vi "Untitled 1.vi"() -> ()   [LabVIEW 2010]
uses:
  <vilib>/MDSplus/Classes/Data_Class/Array_Class/Array.lvclass
  <vilib>/MDSplus/Classes/Data_Class/Array_Class/Float32Array_Class/Float32Array.lvclass
  <vilib>/MDSplus/Classes/Data_Class/Data.lvclass
panel:
  in  "SGL array in":sgl[](array[numeric])
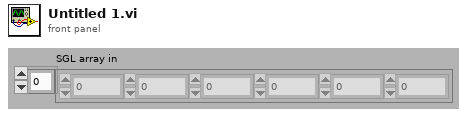
[diagram p1: front panel]
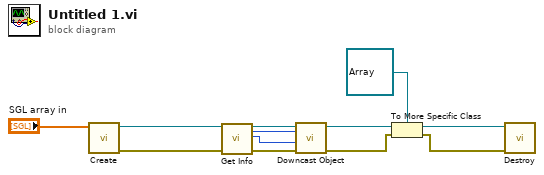
[diagram p0: block diagram]
diagram:
  n1 = call <vilib>:"Create.vi"("SGL array in"="SGL array in") -> ("error out"=w9:errorcluster, "Float32Array out"=w11:refnum<class "Float32Array.lvclass">)  [unwired: 9 in]
  n2 = call-dynamic "Get Info.vi"("Array in"=w11, "error in (no error)"=w9) -> ("Array out"=w10:refnum<class "Float32Array.lvclass">, "Class type out"=w7:u8, "Data type out"=w6:u8, "error out"=w8:errorcluster)  [unwired: 12 in, 2 out]
  n3 = call <vilib>:"Downcast Object.vi"("error in (no error)"=w8, "Data Type"=w6, "Class Type"=w7, "Data in"=w10) -> ("error out"=w3:errorcluster, "Data out"=w5:refnum<class "Data.lvclass">)  [unwired: 6 in]
  n4 = To More Specific Class(target class=refnum<class "Array.lvclass"> refnum ("Array.lvclass"), reference=w5, error in=w3) -> (specific class reference=w4:refnum<class "Array.lvclass">, error out=w2:errorcluster)
  n5 = call-dynamic "Destroy.vi"("error in (no error)"=w2, "Array in"=w4) -> ()  [unwired: 9 in, 1 out]
